vi "BRig_dataTrial_sCue2.vi"() -> (2 "output_sCue2":i32)   [LabVIEW 2014]
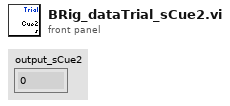
[diagram p1: front panel]
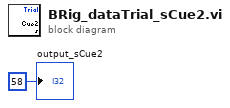
[diagram p0: block diagram]
diagram:
  "output_sCue2" <- 58 ("output_iBlock")
